vi "VCS Set Dc Motor Parameter.vi"(0 "axis in":cluster{"keyHandle":u32, "nodeId":u16}={"keyHandle"=0, "nodeId"=1}, 5 "DC motor parameter":T1, 11 "error in (no error)":errorcluster) -> (4 "axis out":cluster{"keyHandle":u32, "nodeId":u16}={"keyHandle"=0, "nodeId"=1}, 15 "error out":errorcluster)   [LabVIEW 2019, in "maxonEPOS.lvlib"]
doc: "With function <B>VCS_SetDcMotorParameter</B> it is possible to write all DC motor parameters."
uses:
  Examples/maxonEPOS.lvlib
  Resources/EposCmd.dll
  Resources/EposCmd64.dll
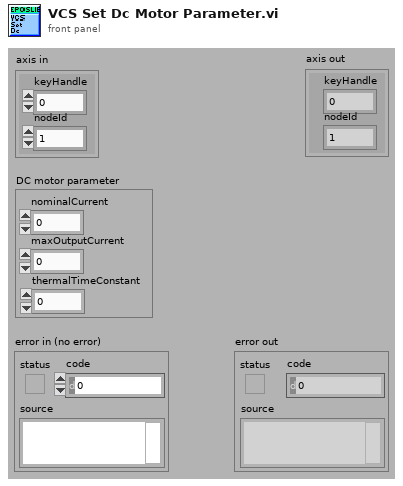
[diagram p1: front panel]
types:
  T1 = cluster{"nominalCurrent":u16, "maxOutputCurrent":u16, "thermalTimeConstant":u16}
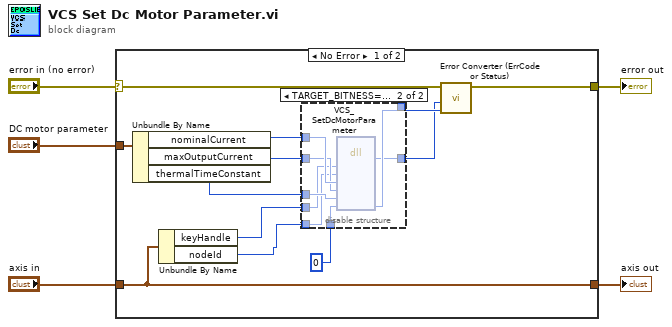
[diagram p0: block diagram]
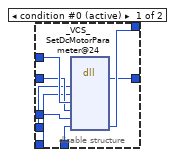
[diagram p2: hidden frame]
diagram:
  n1 = case shown="No Error" "error in (no error)" {
    selector: "error in (no error)" -> [w15 w34]
    tunnel: "axis in" -> [w17 w35]
    tunnel: [w17 w35] -> w4
    tunnel: [w16 w34] -> w3
    tunnel: "DC motor parameter" -> [w13 _]
    frame No Error {
      n2 = Unbundle By Name(w13) -> ("nominalCurrent"=w12:u16, "maxOutputCurrent"=w11:u16, "thermalTimeConstant"=w10:u16)
      n3 = Unbundle By Name(w17) -> ("keyHandle"=w9:u32, "nodeId"=w8:u16)
      n4 = disable-structure shown="TARGET_BITNESS==64" {
        disable-tunnel: u32 0 ("pErrorCode") -> [w25 w33]
        disable-tunnel: w12 -> [w24 w32]
        disable-tunnel: w11 -> [w23 w31]
        disable-tunnel: w10 -> [w22 w30]
        disable-tunnel: w9 -> [w21 w29]
        disable-tunnel: w8 -> [w20 w28]
        disable-tunnel: [w19 w27] -> w7
        disable-tunnel: [w18 w26] -> w6
        frame condition #0 (active) {
          n5 = dll-call lib="C:/workspace/project/scancon/sw/SSI_Tool/InstrumentsInterfaces/Motordriver/maxon EPOS/Resources/EposCmd.*" fn="_VCS_SetDcMotorParameter@24"("KeyHandle"=w21, "NodeId"=w20, "NominalCurrent"=w24, "MaxOutputCurrent"=w23, "ThermalTimeConstant"=w22, "pErrorCode"=w25) -> (w18:i32, "pErrorCode"=w19:u32)  [unwired: 8 in, 2 out]
        }
        frame condition #1 {
          n6 = dll-call lib="C:/Sources/LabView/maxon EPOS/Resources/EposCmd64.*" fn="VCS_SetDcMotorParameter" ("EposCmd.dll:_VCS_SetDcMotorParameter@24")("KeyHandle"=w29, "NodeId"=w28, "NominalCurrent"=w32, "MaxOutputCurrent"=w31, "ThermalTimeConstant"=w30, "pErrorCode"=w33) -> ("Rückgabetyp"=w26:i32, "pErrorCode"=w27:u32)  [unwired: 8 in, 2 out]
        }
      }
      n7 = call "Error Converter (ErrCode or Status).vi"("error code"=w7, "return type"=w6, "error in (no error)"=w15) -> ("error out"=w16:errorcluster)  [unwired: 7 in]
    }
    frame Error {
    }
  }
  "error out" <- w3
  "axis out" <- w4
